vi "Read (Delta Values).vi"(0 "VISA resource name":refnum<visa-resource-name>, 11 "error in (no error)":errorcluster) -> (2 "Checksum Pass":bool, 3 "Timer":u32, 4 "VISA resource name out":refnum<visa-resource-name>, 6 "Delta Angle Vector":sgl[](array[numeric]), 10 "Delta Velocity Vector":sgl[](array[numeric]), 15 "error out":errorcluster)   [LabVIEW 2012, in "MicroStrain 3DM-GXx.lvlib"]
doc: "Read the DeltaAngle Vector and DeltaVelocity Vector."
uses:
  <instrlib>/MicroStrain 3DM-GXx/MicroStrain 3DM-GXx.lvlib
  <instrlib>/MicroStrain 3DM-GXx/Public/Data/Parse Message VIs/Parse (Delta Values).vi
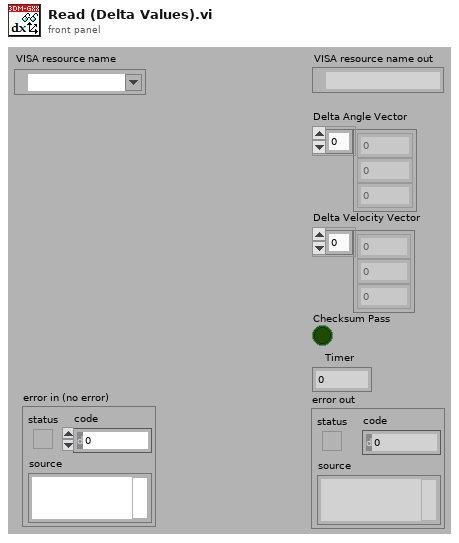
[diagram p1: front panel]
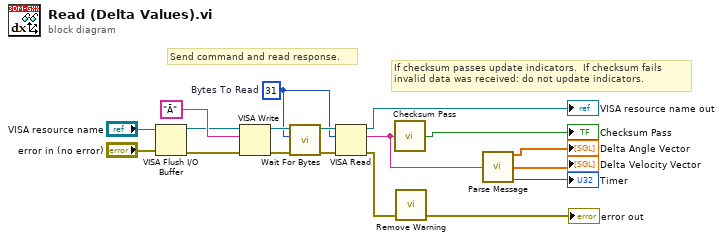
[diagram p0: block diagram]
diagram:
  w13 = u32 31  # Bytes To Read
  # "If checksum passes update indicators.  If checksum fails \ninvalid data was received: do not update indicators."
  # "Send command and read response."
  n1 = VISA Flush I/O Buffer(VISA resource name="VISA resource name", error in (no error)="error in (no error)") -> (VISA resource name out=w2:refnum<visa-resource-name>, error out=w1:errorcluster)  [unwired: 1 in]
  n2 = VISA Write(VISA resource name=w2, write buffer="Ã", error in (no error)=w1) -> (VISA resource name out=w17:refnum<visa-resource-name>, error out=w16:errorcluster)  [unwired: 1 out]
  n3 = call <instrlib>:"Wait For Bytes.vi"("error in (no error)"=w16, "Bytes To Read (0)"=w13, "VISA resource name"=w17) -> ("error out"=w15:errorcluster, "VISA resource name out"=w14:refnum<visa-resource-name>)  [unwired: 7 in]
  n4 = VISA Read(VISA resource name=w14, byte count=w13, error in (no error)=w15) -> (VISA resource name out=→"VISA resource name out":refnum<visa-resource-name>, read buffer=w12:string, error out=w9:errorcluster)  [unwired: 1 out]
  n5 = call <instrlib>:"Checksum Pass.vi"("Message In"=w12) -> ("Checksum Pass"=→"Checksum Pass":bool)  [unwired: 4 in]
  n6 = call <instrlib>:"Remove Warning.vi"("error in (no error)"=w9) -> ("error out"=→"error out":errorcluster)  [unwired: 3 in, 1 out]
  n7 = call-poly <instrlib>:"Parse Message.vi"("Message In"=w12) -> ("DeltaAngleVector"=→"Delta Angle Vector":sgl[], "DeltaVelocityVector"=→"Delta Velocity Vector":sgl[], "Timer"=→"Timer":u32)  [unwired: 12 in]
